vi "Analog Window Comparison.vi"(0 "Upper Level":dbl, 2 "Condition":enum16{"Inside Window", "Outside Window"}(ring), 5 "Lower Level":dbl, 7 "Data":dbl, 11 "error in":errorcluster) -> (4 "Result":bool, 15 "error out":errorcluster)   [LabVIEW 2010]
doc: "This VI does basic analog window comparisons on the Data input."
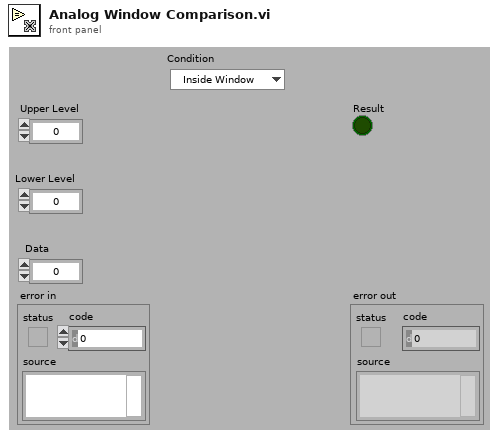
[diagram p1: front panel]
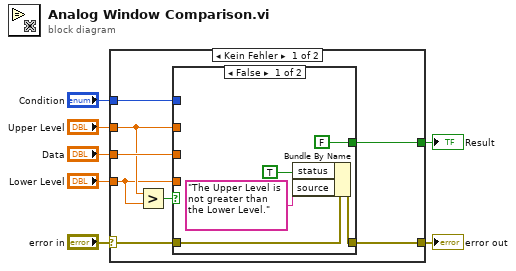
[diagram p0: block diagram]
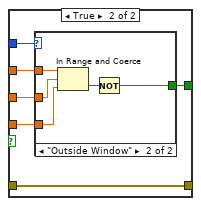
[diagram p2: hidden frame]
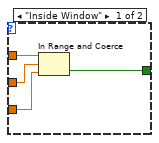
[diagram p3: hidden frame]
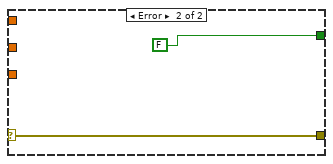
[diagram p4: hidden frame]
diagram:
  n1 = case shown="Kein Fehler" "error in" {
    selector: "error in" -> [w9 w37]
    tunnel: [w8 w37] -> w6
    tunnel: "Condition" -> [w15 _]
    tunnel: "Data" -> [w14 _]
    tunnel: "Lower Level" -> [w11 _]
    tunnel: [w13 FALSE] -> w2
    tunnel: "Upper Level" -> [w12 _]
    frame No Error {
      n2 = Greater?(x=w12, y=w11) -> (0:w10:bool)
      n3 = case shown="FALSE" w10 {
        tunnel: w15 -> [_ w26]
        tunnel: w14 -> [_ w25]
        tunnel: [FALSE w24] -> w13
        tunnel: w12 -> [_ w23]
        tunnel: w11 -> [_ w22]
        tunnel: w9 -> [w19 w21]
        tunnel: [w18 w21] -> w8
        frame False {
          n4 = Bundle By Name(cluster=w19, "status"=TRUE, "source"="The Upper Level is not greater than the Lower Level.") -> (w18:errorcluster)
        }
        frame True {
          n5 = case shown="\"Outside Window\"" w26 {
            tunnel: w23 -> [w30 w35]
            tunnel: w25 -> [w29 w34]
            tunnel: w22 -> [w28 w33]
            tunnel: [w27 w31] -> w24
            frame "Inside Window" {
              n6 = In Range and Coerce(upper limit=w30, x=w29, lower limit=w28) -> (In Range?=w27:bool)  [unwired: 1 out]
            }
            frame "Outside Window" {
              n7 = In Range and Coerce(upper limit=w35, x=w34, lower limit=w33) -> (In Range?=w32:bool)  [unwired: 1 out]
              n8 = Not(x=w32) -> (.not. x?=w31:bool)
            }
          }
        }
      }
    }
    frame Error {
    }
  }
  "error out" <- w6
  "Result" <- w2
